vi "Save for Previous.vi"(8 "error in (no error)":errorcluster, 10 "File Path":path, 11 "Session in":refnum<class "Session.lvclass">) -> (0 "error out":errorcluster, 3 "Session out":refnum<class "Session.lvclass">)   [LabVIEW 2020, in "Save for Previous Version.lvlib" / "Session.lvclass"]
uses:
  Session.lvclass
  LabVIEW File/LabVIEW File.lvclass
  \\Mac\Home/JKI/GitHub/vipm-io/a-version-explorer-for-labview/experiments/save-for-previous-version/source/File/File.lvclass/File.lvclass
  Session.lvclass/Session.ctl
  <userlib>/_OpenG.lib/file/file.llb/Append Path to Root if Relative - Scalar__ogtk.vi
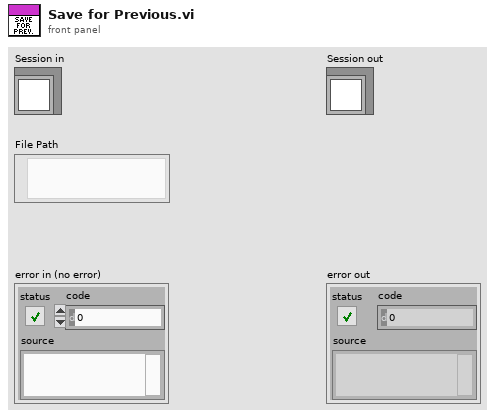
[diagram p1: front panel]
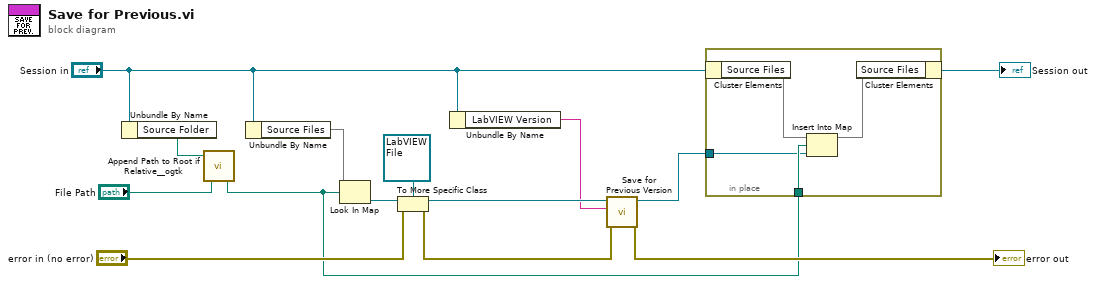
[diagram p0: block diagram]
diagram:
  n1 = Unbundle By Name("Session in") -> ("Source Folder"=w6:path)
  n2 = call-poly <userlib>:"Append Path to Root if Relative__ogtk.vi"("Absolute or Relative Path"="File Path", "Root Path"=w6) -> ("Absolute or Appended Path"=w4:path)
  n3 = Unbundle By Name("Session in") -> ("Source Files"=w14:map{path, refnum<class "File.lvclass">})
  n4 = Look In Map(map=w14, key=w4) -> (value=w13:refnum<class "File.lvclass">)  [unwired: 1 in, 1 out]
  n5 = To More Specific Class(target class=refnum<class "LabVIEW File.lvclass"> refnum ("LabVIEW File in"), reference=w13, error in="error in (no error)") -> (specific class reference=w12:refnum<class "LabVIEW File.lvclass">, error out=w8:errorcluster)
  n6 = Unbundle By Name("Session in") -> ("LabVIEW Version"=w7:string)
  n7 = call-dynamic "Save for Previous Version.vi"("error in (no error)"=w8, "LabVIEW Version"=w7, "LabVIEW File in"=w12) -> ("error out"=→"error out":errorcluster, "LabVIEW File out"=w3:refnum<class "LabVIEW File.lvclass">)  [unwired: 5 in, 2 out]
  n8 = in-place {
    in-place-border: w4 -> [w16]
    in-place-border: w3 -> [w15]
    n9 = in-place-cluster #1("Session in") -> ("Source Files"=w18:map{path, refnum<class "File.lvclass">})
    n10 = Insert Into Map(map in=w18, key=w16, value=w15) -> (map out=w17:map{path, refnum<class "File.lvclass">})  [unwired: 2 out]
    n11 = in-place-cluster #1("Source Files"=w17) -> (→"Session out":refnum<class "Session.lvclass">)
  }
